vi "Create Type Descriptor Map.vi"(8 "error in (no error)":errorcluster, 11 "TwinCAT ADS in":refnum<class "TwinCAT ADS.lvclass">) -> (0 "error out":errorcluster, 3 "TwinCAT ADS out":refnum<class "TwinCAT ADS.lvclass">)   [LabVIEW 2018, in "TwinCAT ADS.lvclass"]
uses:
  TwinCAT ADS.lvclass
  TwinCAT ADS.lvclass/TwinCAT ADS.ctl
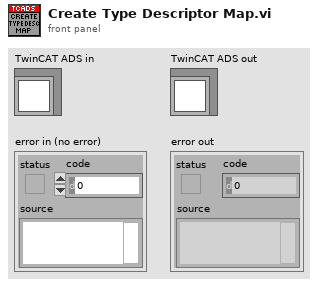
[diagram p1: front panel]
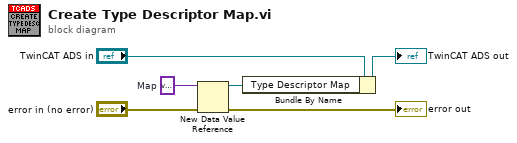
[diagram p0: block diagram]
diagram:
  w4 = variant  # Map
  n1 = New Data Value Reference(data value=w4, error in="error in (no error)") -> (data value reference=w2:refnum<data-value>, error out=→"error out":errorcluster)
  n2 = Bundle By Name(cluster="TwinCAT ADS in", "Type Descriptor Map"=w2) -> (→"TwinCAT ADS out":refnum<class "TwinCAT ADS.lvclass">)
